vi "ClientSrv Server Runlevels_srv.vi"(0 "method":T1, 7 "certificate":string, 11 "runlevel/bootmode":string) -> (4 "names":string[](array[string]), 8 "current":string, 15 "error out":errorcluster)   [LabVIEW 2012]
uses:
  typedefs/t_ClientSrv Server Runlevels Methods.ctl
  typedefs/t_ClientSrv Access Levels.ctl
  typedefs/t_ClientSrv Runlevels Methods.ctl
  luaview/typedefs/t_LuaVIEW Task List Methods.ctl
  library/glb_Library Configuration Globals.vi
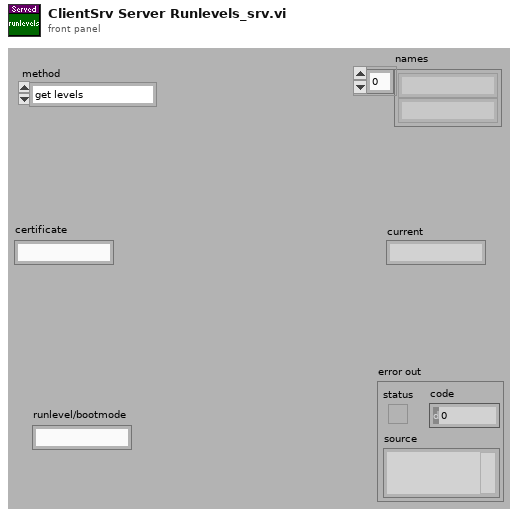
[diagram p1: front panel]
types:
  T1 = typedef "t_ClientSrv Server Runlevels Methods.ctl" = enum16{"get levels", "get modes", "change", "set bootmode"}
  T2 = typedef "t_ClientSrv Access Levels.ctl" = enum16{"observer", "operator", "local"}
  T3 = typedef "t_ClientSrv Runlevels Methods.ctl" = enum16{"initialize", "get path", "get levels", "get modes", "set current", "cleanup"}
  T4 = typedef "t_LuaVIEW Task List Methods.ctl" = enum16{"clear list", "add", "test", "remove", "get ref", "get task info", "get list", "get script info", "ongoing?", "resume", "pause", "stop", "confirm", "message"}
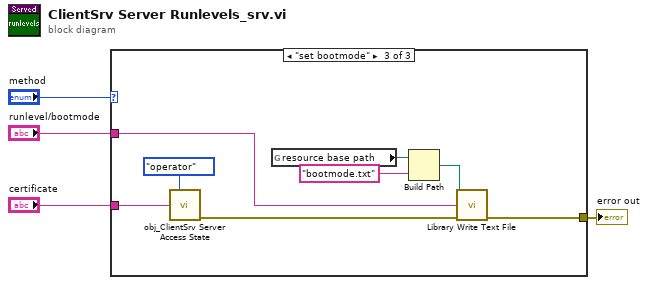
[diagram p0: block diagram]
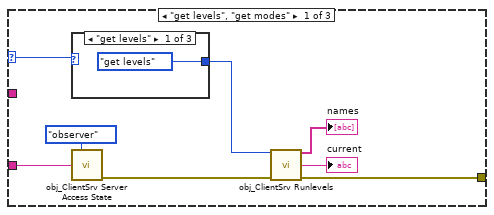
[diagram p2: hidden frame]
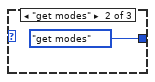
[diagram p3: hidden frame]
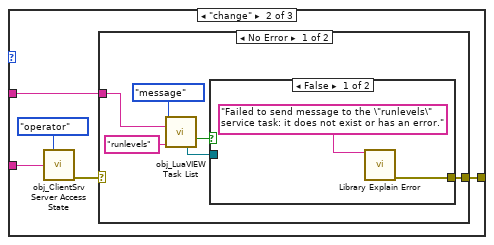
[diagram p5: hidden frame]
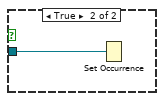
[diagram p6: hidden frame]
diagram:
  n1 = case shown="\"set bootmode\"" "method" {
    selector: "method" -> [w5 _ _]
    tunnel: [w12 w16 w35] -> w4
    tunnel: "certificate" -> [w7 w18 w36]
    tunnel: "runlevel/bootmode" -> [_ w15 w31]
    frame "get levels", "get modes" {
      n2 = case shown="\"get levels\"" w5 {
        tunnel: [t_ClientSrv_Runlevels_Methods."get levels" ("method") t_ClientSrv_Runlevels_Methods."get modes" ("method") _] -> w11
        frame "get levels" {
        }
        frame "get modes" {
        }
        frame Default {
        }
      }
      n3 = call "obj_ClientSrv Server Access State.vi"("access level"=t_ClientSrv_Access_Levels."observer", "certificate in"=w7) -> ("error out"=w8:errorcluster)  [unwired: 11 in, 2 out]
      n4 = call "obj_ClientSrv Runlevels.vi"("method"=w11, "error in (no error)"=w8) -> ("names"=→"names":string[], "current"=→"current":string, "error out"=w12:errorcluster)  [unwired: 10 in, 1 out]
    }
    frame "change" {
      n5 = call "obj_ClientSrv Server Access State.vi"("access level"=t_ClientSrv_Access_Levels."operator", "certificate in"=w18) -> ("error out"=w17:errorcluster)  [unwired: 11 in, 2 out]
      n6 = case shown="No Error" w17 {
        selector: w17 -> [_ w29]
        tunnel: [w25 w29] -> w16
        tunnel: w15 -> [w20 _]
        frame No Error {
          n7 = call "obj_LuaVIEW Task List.vi"("method"=t_LuaVIEW_Task_List_Methods."message", "message"=w20, "task identifier"="runlevels") -> ("set/ongoing"=w24:bool, "wakeup occurrence"=w23:refnum<k4>)  [unwired: 7 in, 4 out]
          n8 = case shown="False" w24 {
            tunnel: [w27 _] -> w25
            tunnel: w23 -> [_ w28]
            frame False {
              n9 = call "Library Explain Error.vi"("explanation prefix (none)"="Failed to send message to the \"runlevels\" service task: it does not exist or has an error." ("format string")) -> ("explained error"=w27:errorcluster)  [unwired: 14 in]
            }
            frame True {
              n10 = Set Occurrence(w28) -> ()
            }
          }
        }
        frame Error {
        }
      }
    }
    frame "set bootmode" {
      n11 = call "obj_ClientSrv Server Access State.vi"("access level"=t_ClientSrv_Access_Levels."operator", "certificate in"=w36) -> ("error out"=w30:errorcluster)  [unwired: 11 in, 2 out]
      n12 = global read "glb_Library Configuration Globals.vi" "resource base path"() -> (w34:path)
      n13 = Build Path(base path=w34, name or relative path="bootmode.txt") -> (appended path=w32:path)
      n14 = call "Library Write Text File.vi"("file path"=w32, "text to write"=w31, "error in (no error)"=w30) -> ("error out"=w35:errorcluster)  [unwired: 11 in, 1 out]
    }
  }
  "error out" <- w4
